vi "NIMS_DF_fir_halfband(m, f, ripple,k,h).vi"(7 "type":enum32{"high"}(ring), 8 "method":enum32{"kaiser"}(ring), 9 "ripple":dbl, 10 "f":dbl, 11 "flag":enum32{"minorder"}(ring)) -> (0 "error":i32, 3 "b":dbl[](array[numeric]))   [LabVIEW 2017, in "NI_DigFilter_MathScript.lvlib"]
uses:
  <vilib>/addons/Digital Filter Design/NI_DigFilter_MathScript.lvlib
  <vilib>/addons/Digital Filter Design/NI_DigFilterLicensed.lvlib
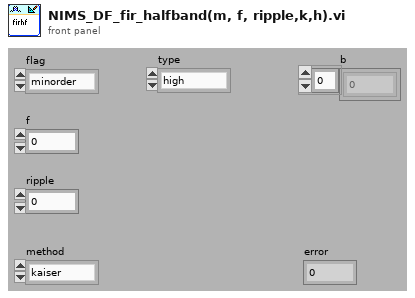
[diagram p1: front panel]
types:
  T1 = typedef "NI_DigFilterLicensed.lvlib/DFD Multirate Filter Obj.ctl" = cluster{"mMRate_Structure":enum16{"CIC", "FIR", "IIR", "Lattice"}, "mMRate_Mode":T2, "mMRate_Factor":i32, "mMRate_FIRParams":cluster{"mMRate_FIR_H":dbl[], "mMRate_FIR_IsNyquist?":bool, "mMRate_FIR_IsSymmetric?":bool}, "mMRate_CICParams":cluster{"mMRate_CIC_#Stage":i32, "mMRate_CIC_Lag":i32, "mMRate_CIC_Type":enum16{"Lowpass", "Highpass"}}, "mMRate_Order":i32, "mMRate_Version":string, "mMRate_Comments":string, "mMRate_RationalFactor":cluster{"mMRate_L":i32, "mMRate_M":i32}, "mMRate_Fs":dbl, "mMRate_Quantized?":bool, "mMRate_QFilterGain":dbl, "mMRate_CoefWl":i16, "mMRate_Scaling":cluster{"mMRate_ScaleByPowerOf2?":bool, "mMRate_ScaleType":T3}, "mMRate_InputWl":i16, "mMRate_OutputWl":i16, "mMRate_OutputMode":T4, "mMRate_MultMode":T5, "mMRate_BitPruning":bool, "mMRate_GainWl":i16, "mMRate_OutputFwl":i16, "mMRate_SumIwl":i16, "mMRate_InputIwl ":i16, "mMRate_SumWl":i16, "mMRate_CoefIwl":i16}
  T2 = typedef "NI_DigFilterLicensed.lvlib/DFD Multirate Mode.ctl" = i16
  T3 = typedef "NI_DigFilterLicensed.lvlib/DFD Coef Norm Type.ctl" = enum16{"No Norm", "Time Domain 1-Norm", "Time Domain 2-Norm", "Time Domain Inf-Norm"}
  T4 = typedef "NI_DigFilterLicensed.lvlib/DFD Round-off Mode.ctl" = enum16{"Nearest", "Truncation"}
  T5 = typedef "NI_DigFilterLicensed.lvlib/DFD FXP MRate Multiply Mode.ctl" = enum16{"Truncated", "Full"}
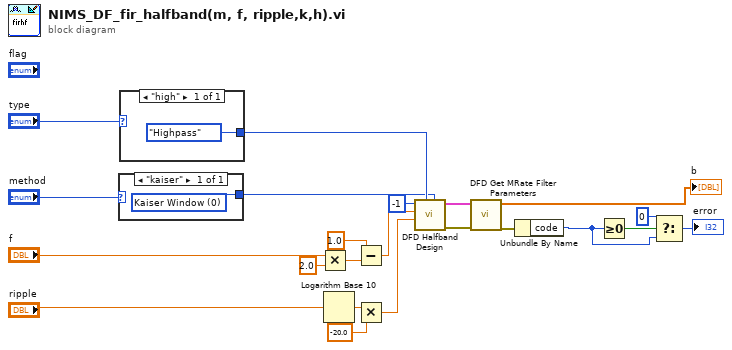
[diagram p0: block diagram]
diagram:
  n1 = case shown="\"kaiser\"" "method" {
    tunnel: [w23] -> w8
    frame "kaiser" {
      w23 = u16 0 items=["Kaiser Window", "Dolph-Chebyshev Window", "Equi-Ripple", "Positive Equi-Ripple", "Max Flat"] ("method")
    }
  }
  n2 = case shown="\"high\"" "type" {
    tunnel: [enum16{"Lowpass", "Highpass"}."Highpass" ("filter type")] -> w12
    frame "high" {
    }
  }
  n3 = Multiply(x="f", y=2.0) -> (x*y=w15:dbl)
  n4 = Logarithm Base 10(1:"ripple") -> (0:w19:dbl)
  n5 = Subtract(x=1.0, y=w15) -> (x-y=w13:dbl)
  n6 = Multiply(x=w19, y=-20.0) -> (x*y=w17:dbl)
  n7 = call <vilib>:"DFD Halfband Design.vi"("method"=w8, "filter type"=w12, "stopband attenuation [dB]"=w17, "roll off"=w13, "order"=-1) -> ("error out"=w20:errorcluster, "multirate filter out"=w21:T1)  [unwired: 3 in, 2 out]
  n8 = call <vilib>:"DFD Get MRate Filter Parameters.vi"("error in (no error)"=w20, "multirate filter in"=w21) -> ("error out"=w5:errorcluster, "h(n)"=→"b":dbl[])  [unwired: 1 in, 7 out]
  n9 = Unbundle By Name(w5) -> ("code"=w2:i32)
  n10 = Greater Or Equal To 0?(x=w2) -> (x >= 0?=w4:bool)
  n11 = Select(t=0 ("error"), s=w4, f=w2) -> (s? t:f=→"error":i32)
